vi "Set Logging Root.vi"(8 "error in (no error)":errorcluster, 10 "Logging Root":path, 11 "EventAPI in":refnum<class "EventAPI.lvclass">) -> (0 "error out":errorcluster, 3 "EventAPI out":refnum<class "EventAPI.lvclass">)   [LabVIEW 2020, in "Volatus.lvlib" / "EventAPI.lvclass"]
uses:
  EventAPI.lvclass
  EventAPI.lvclass/EventAPI.ctl
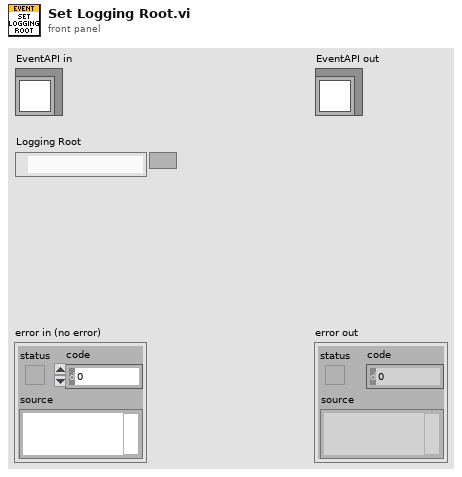
[diagram p1: front panel]
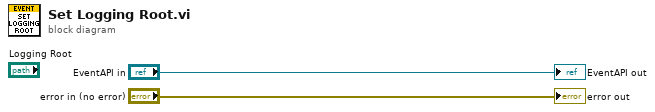
[diagram p0: block diagram]
diagram:
  "error out" <- "error in (no error)"
  "EventAPI out" <- "EventAPI in"
